vi "MUSIQC_trap_control_trap2.vi"() -> ()   [LabVIEW 2012]
uses:
  <vilib>/DAQmx/read.llb/DAQmx Read (Counter U32 1Chan 1Samp).vi
  <vilib>/DAQmx/create/channels.llb/DAQmx Create Channel (CO-Pulse Generation-Frequency).vi
  <vilib>/DAQmx/configure/timing.llb/DAQmx Timing (Implicit).vi
  <vilib>/DAQmx/create/channels.llb/DAQmx Create Channel (CI-Count Edges).vi
  <vilib>/DAQmx/configure/timing.llb/DAQmx Timing (Sample Clock).vi
  oven_state_global.vi
  <vilib>/Analysis/baseanly.llb/Mean (DBL).vi
  <vilib>/DAQmx/miscellaneous.llb/DAQmx Fill In Error Info.vi
  <vilib>/Utility/file.llb/Write To Spreadsheet File (I64).vi
  <resource>/objmgr/daqmx.rc
  <vilib>/Analysis/NI_AALBase.lvlib
panel:
  in  "Tsunami":bool
  in  "Oven":bool
  in  "Orange":bool
  in  "Sample rate":dbl=50.0 format="%0.2f"
  in  "snap":bool
  in  "Threshold":u32
  in  "Auto Load":bool
  in  "RF":bool
  in  "Blue":bool
  in  "Red":bool
  out "Mean/Variance":dbl
  out "Variance":dbl format="%0.2f"
  out "Mean":dbl format="%0.2f"
  in  "Samples per averaging\nblock":i32=100 min=1 step=1
  in  "stop":bool
  out "PMT Counts":cluster{"mean":dbl, u32}(graph)
  out "Counts total":dbl
  # "Trap 2"
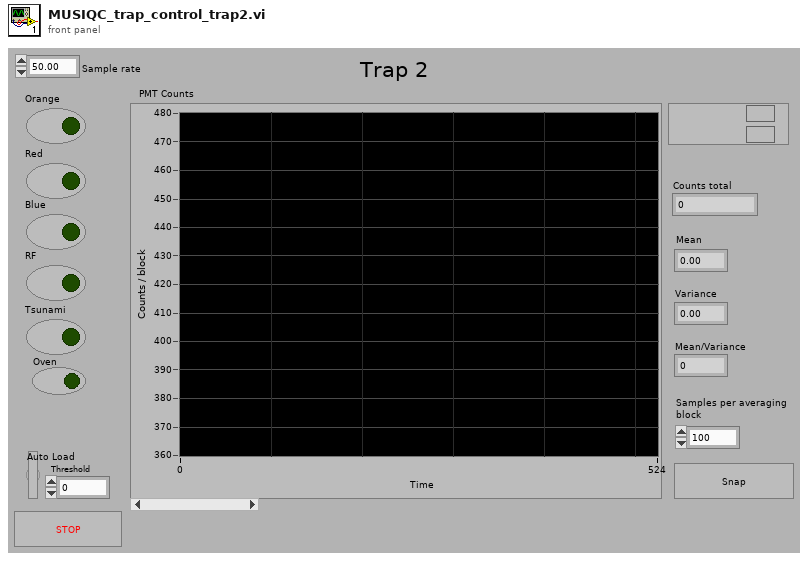
[diagram p1: front panel]
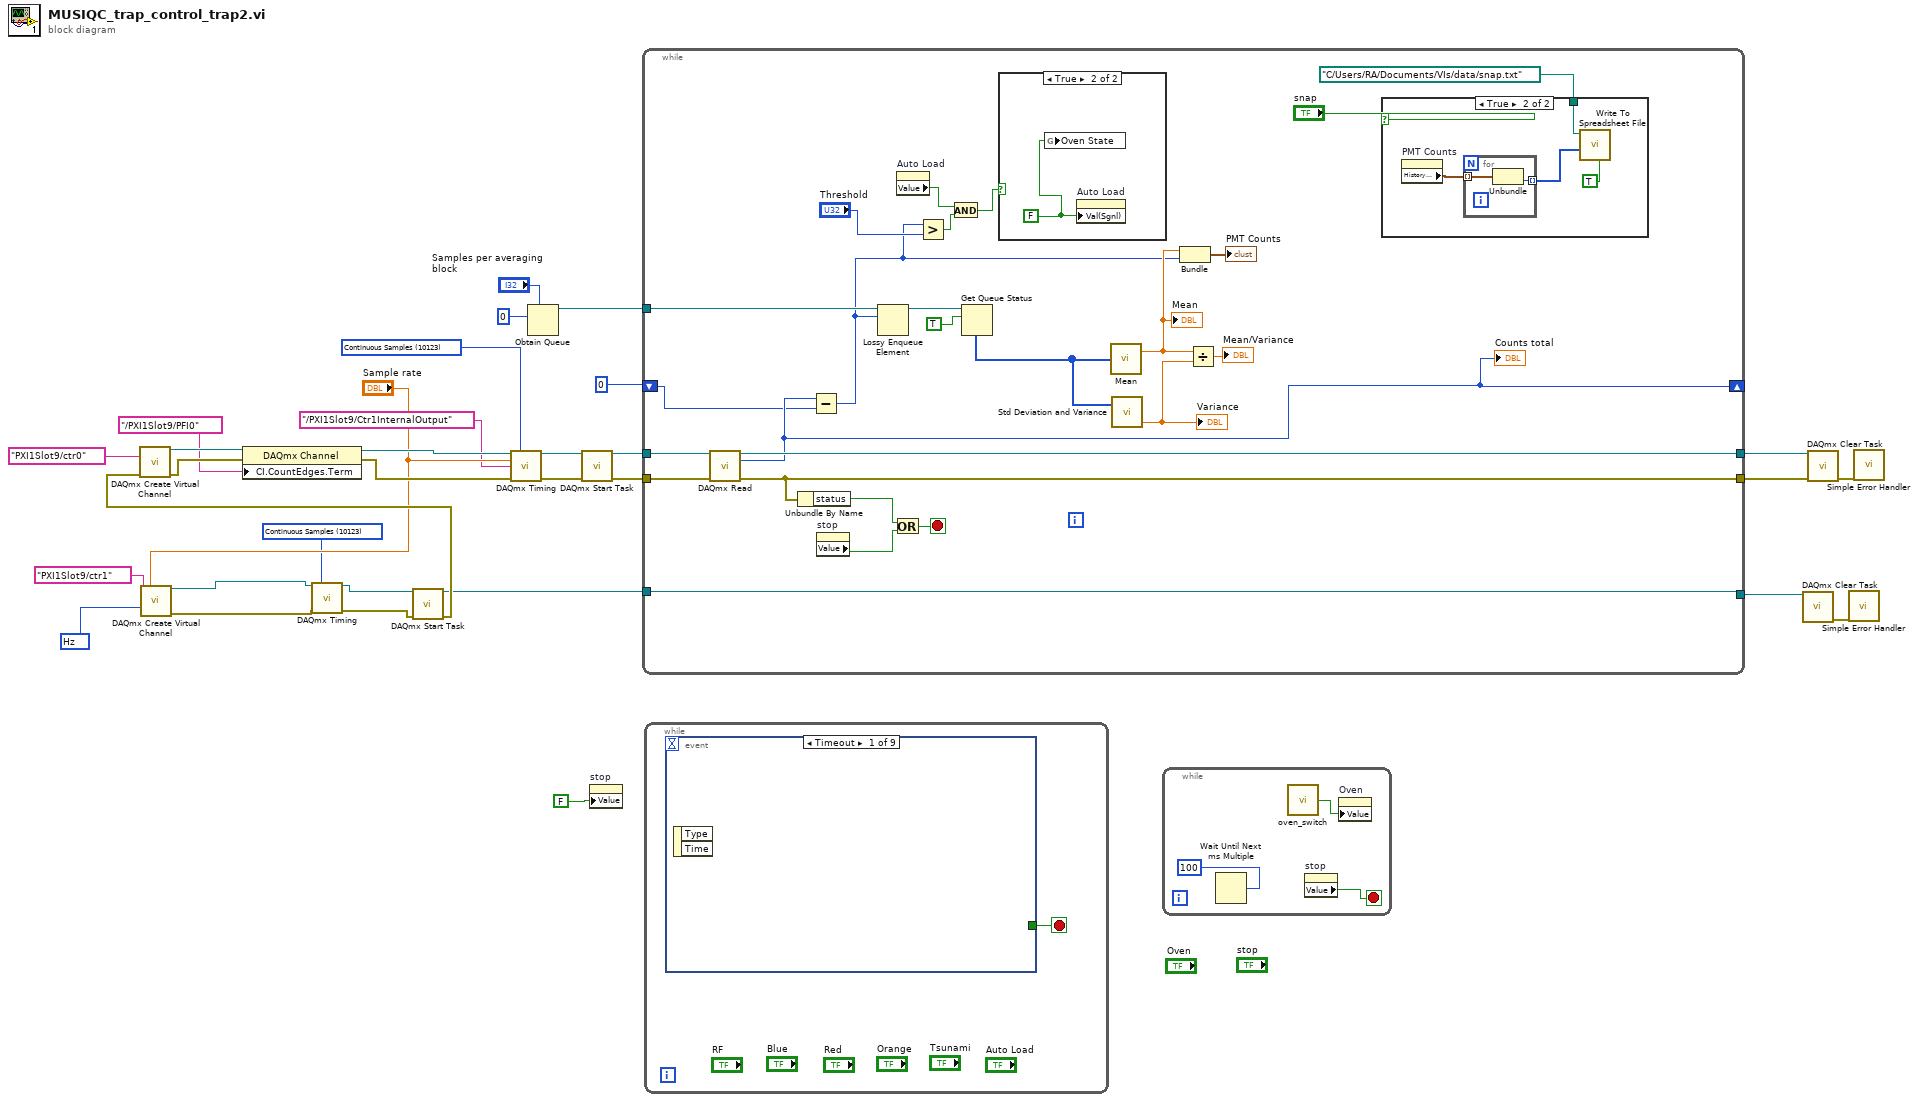
[diagram p0: block diagram]
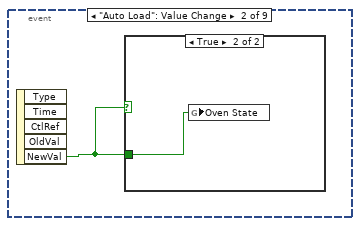
[diagram p2: hidden frame]
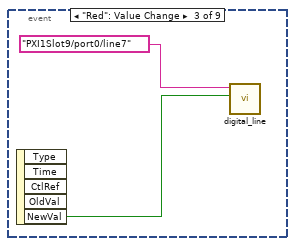
[diagram p4: hidden frame]
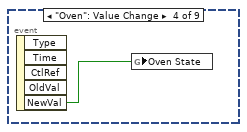
[diagram p5: hidden frame]
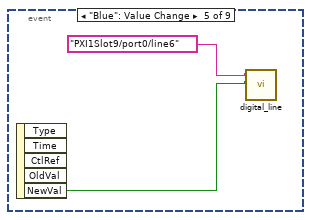
[diagram p6: hidden frame]
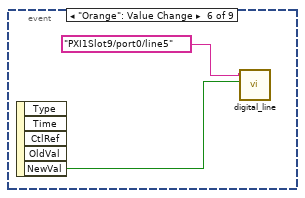
[diagram p7: hidden frame]
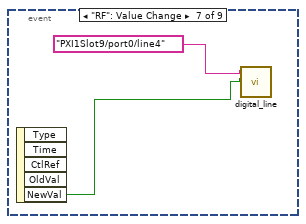
[diagram p8: hidden frame]
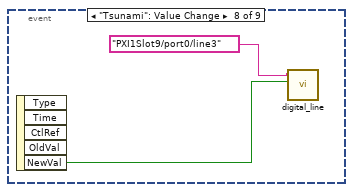
[diagram p9: hidden frame]
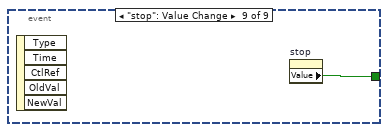
[diagram p10: hidden frame]
diagram:
  w1 = 10123 items=["Finite Samples"=10178, "Continuous Samples"=10123, "Hardware Timed Single Point"=12522] ("sample mode")
  w9 = 10373 items=["Hz"=10373] ("units")
  w15 = 10123 items=["Finite Samples"=10178, "Continuous Samples"=10123, "Hardware Timed Single Point"=12522] ("sample mode")
  n1 = call-poly <vilib>:"DAQmx Create Virtual Channel.vi"("frequency"="Sample rate", "counter"=tag "PXI1Slot9/ctr1", "units"=w9) -> ("task out"=w5:refnum<k21>, "error out"=w4:errorcluster)  [unwired: 11 in]
  n2 = call-poly <vilib>:"DAQmx Timing.vi"("task/channels in"=w5, "sample mode"=w1, "error in"=w4) -> ("task out"=w3:refnum<k21>, "error out"=w2:errorcluster)  [unwired: 11 in]
  n3 = call <vilib>:"DAQmx Start Task.vi"("task/channels in"=w3, "error in"=w2) -> ("task out"=w12:refnum<k21>, "error out"=w13:errorcluster)  [unwired: 12 in]
  n4 = call-poly <vilib>:"DAQmx Create Virtual Channel.vi"("counter"=tag "PXI1Slot9/ctr0", "error in"=w13) -> ("task out"=w23:refnum<k21>, "error out"=w22:errorcluster)  [unwired: 12 in]
  n5 = property class="DAQmx Channel"(reference=w23, error in=w22, "CI.CountEdges.Term"=tag "/PXI1Slot9/PFI0") -> (reference out=w25:refnum<k21>, error out=w24:errorcluster)
  n6 = call-poly <vilib>:"DAQmx Timing.vi"("task/channels in"=w25, "sample mode"=w15, "rate"="Sample rate", "source"=tag "/PXI1Slot9/Ctr1InternalOutput", "error in"=w24) -> ("task out"=w31:refnum<k21>, "error out"=w30:errorcluster)  [unwired: 9 in]
  n7 = Obtain Queue(max queue size (-1, unlimited)="Samples per averaging\nblock", element data type=u32 0) -> (queue out=w18:refnum<queue>)  [unwired: 3 in, 2 out]
  n8 = call <vilib>:"DAQmx Start Task.vi"("task/channels in"=w31, "error in"=w30) -> ("task out"=w26:refnum<k21>, "error out"=w8:errorcluster)  [unwired: 12 in]
  n9 = property on="stop" class="Bool (strict)"("Value"=FALSE ("stop")) -> ()  [unwired: 2 in, 2 out]
  n10 = while {
    shift-right: [w38] -> _
    shift-left: u32 0 -> [w37]
    tunnel: [w55] -> w28
    tunnel: [w54] -> w27
    tunnel: w26 -> [w53]
    tunnel: w18 -> [w52]
    tunnel: w12 -> [w34]
    tunnel: [w34] -> w10
    tunnel: w8 -> [w33]
    stop <- w57 stop-if-true
    n11 = call-poly <vilib>:"DAQmx Read.vi"("task/channels in"=w53, "error in"=w33) -> ("task out"=w54:refnum<k21>, "data"=w38:u32, "error out"=w55:errorcluster)  [unwired: 11 in]
    "Counts total" <- w38
    n12 = Unbundle By Name(w55) -> ("status"=w56:bool)
    n13 = Subtract(x=w38, y=w37) -> (x-y=w36:u32)
    n14 = property on="stop" class="Bool (strict)"() -> ("Value"=w46:bool)  [unwired: 2 in, 2 out]
    n15 = Lossy Enqueue Element(queue=w52, element=w36) -> (queue out=w51:refnum<queue>)  [unwired: 1 in, 3 out]
    n16 = Or(x=w56, y=w46) -> (x .or. y?=w57:bool)
    n17 = property on="Auto Load" class="Bool (strict)"() -> ("Value"=w43:bool)  [unwired: 2 in, 2 out]
    n18 = Greater?(x=w36, y="Threshold") -> (0:w44:bool)
    n19 = And(x=w43, y=w44) -> (x .and. y?=w42:bool)
    n20 = Get Queue Status(queue=w51, return elements? (F)=TRUE) -> (elements=w40:u32[])  [unwired: 1 in, 7 out]
    n21 = case shown="True" w42 {
      frame False {
      }
      frame True {
        w64 = FALSE ("Auto Load")
        n22 = global write "oven_state_global.vi" "Oven State"(w64) -> ()
        n23 = property on="Auto Load" class="Bool (strict)"("Val(Sgnl)"=w64) -> ()  [unwired: 2 in, 2 out]
      }
    }
    n24 = call-poly <vilib>:"Mean.vi"("X"=w40) -> ("mean"=w47:dbl)  [unwired: 1 out]
    "Mean" <- w47
    n25 = call <vilib>:"Std Deviation and Variance.vi"("X"=w40) -> ("variance"=w49:dbl)  [unwired: 1 in, 2 out]
    "Variance" <- w49
    n26 = Bundle("mean"=w47, w36) -> (→"PMT Counts":cluster{"mean":dbl, u32})  [unwired: 1 in]
    n27 = Divide(x=w47, y=w49) -> (x/y=→"Mean/Variance":dbl)
    n28 = case shown="True" "snap" {
      tunnel: path "C:/Users/RA/Documents/VIs/data/snap.txt" ("file path (dialog if empty)") -> [_ w60]
      frame False {
      }
      frame True {
        n29 = property on="PMT Counts" class="WFChart (strict)"() -> ("History Data"=w59:cluster{"mean":dbl, u32}[])  [unwired: 2 in, 2 out]
        n30 = for {
          tunnel: w59 -> [w63] mode=indexing
          tunnel: [w62] -> w58 mode=indexing
          n31 = Unbundle(w63) -> (w62:u32)  [unwired: 1 out]
        }
        n32 = call-poly <vilib>:"Write To Spreadsheet File.vi"("transpose? (no:F)"=TRUE, "1D data"=w58, "file path (dialog if empty)"=w60) -> ()  [unwired: 5 in, 1 out]
      }
    }
  }
  n33 = while {
    stop <- w65 stop-if-true
    n34 = event shown="[0] Timeout" {
      selector: _ -> [_ _ _ _ _ _ _ _ _]
      dyn-events: _ -> [_ _ _ _ _ _ _ _ _]
      timeout: _ -> [_ _ _ _ _ _ _ _ _]
      tunnel: [_ _ _ _ _ _ _ _ w79] -> w65
      event Timeout {
        n35 = event-data() -> ()  [unwired: 1 in, 2 out]
      }
      event "Auto Load": Value Change {
        n36 = event-data() -> ("NewVal"=w66:bool)  [unwired: 1 in, 4 out]
        n37 = case shown="True" w66 {
          tunnel: w66 -> [_ w67]
          frame False {
          }
          frame True {
            n38 = global write "oven_state_global.vi" "Oven State"(w67) -> ()
          }
        }
      }
      event "Red": Value Change {
        n39 = event-data() -> ("NewVal"=w68:bool)  [unwired: 1 in, 4 out]
        n40 = call "digital_line.vi"("NewVal"=w68, "lines"=tag "PXI1Slot9/port0/line7") -> ()  [unwired: 2 in]
      }
      event "Oven": Value Change {
        n41 = event-data() -> ("NewVal"=w70:bool)  [unwired: 1 in, 4 out]
        n42 = global write "oven_state_global.vi" "Oven State"(w70) -> ()
      }
      event "Blue": Value Change {
        n43 = event-data() -> ("NewVal"=w71:bool)  [unwired: 1 in, 4 out]
        n44 = call "digital_line.vi"("NewVal"=w71, "lines"=tag "PXI1Slot9/port0/line6") -> ()  [unwired: 2 in]
      }
      event "Orange": Value Change {
        n45 = event-data() -> ("NewVal"=w73:bool)  [unwired: 1 in, 4 out]
        n46 = call "digital_line.vi"("NewVal"=w73, "lines"=tag "PXI1Slot9/port0/line5") -> ()  [unwired: 2 in]
      }
      event "RF": Value Change {
        n47 = event-data() -> ("NewVal"=w75:bool)  [unwired: 1 in, 4 out]
        n48 = call "digital_line.vi"("NewVal"=w75, "lines"=tag "PXI1Slot9/port0/line4") -> ()  [unwired: 2 in]
      }
      event "Tsunami": Value Change {
        n49 = event-data() -> ("NewVal"=w77:bool)  [unwired: 1 in, 4 out]
        n50 = call "digital_line.vi"("NewVal"=w77, "lines"=tag "PXI1Slot9/port0/line3") -> ()  [unwired: 2 in]
      }
      event "stop": Value Change {
        n51 = event-data() -> ()  [unwired: 1 in, 5 out]
        n52 = property on="stop" class="Bool (strict)"() -> ("Value"=w79:bool)  [unwired: 2 in, 2 out]
      }
    }
  }
  n53 = while {
    stop <- w80 stop-if-true
    n54 = Wait Until Next ms Multiple(millisecond multiple=u32 100) -> ()  [unwired: 1 out]
    n55 = call "oven_switch.vi"() -> ("Final state"=w82:bool)  [unwired: 2 in]
    n56 = property on="stop" class="Bool (strict)"() -> ("Value"=w80:bool)  [unwired: 2 in, 2 out]
    n57 = property on="Oven" class="Bool (strict)"("Value"=w82) -> ()  [unwired: 2 in, 2 out]
  }
  n58 = call <vilib>:"DAQmx Clear Task.vi"("task in"=w10) -> ("error out"=w11:errorcluster)  [unwired: 14 in]
  n59 = call <vilib>:"DAQmx Clear Task.vi"("task in"=w27, "error in"=w28) -> ("error out"=w16:errorcluster)  [unwired: 13 in]
  n60 = call <vilib>:"Simple Error Handler.vi"("error in (no error)"=w11) -> ()  [unwired: 4 in, 5 out]
  n61 = call <vilib>:"Simple Error Handler.vi"("error in (no error)"=w16) -> ()  [unwired: 4 in, 5 out]
